vi "V_1.vi"() -> ()   [LabVIEW 2014]
uses:
  <vilib>/LabVIEW Interface for Arduino/Type Defs/Board Type.ctl
  <vilib>/LabVIEW Interface for Arduino/Type Defs/Connection Type.ctl
  <vilib>/LabVIEW Interface for Arduino/Type Defs/Pin Mode.ctl
  <vilib>/LabVIEW Interface for Arduino/LabVIEW Interface for Arduino.lvlib
panel:
  in  "Left":bool caption="Right"
  in  "Right":bool
  in  "VISA resource":refnum<visa-resource-name>
  in  "?":bool
  in  "Forward":bool
  in  "Backward":bool
  in  "Dial":dbl(knob) scale=0.0..255.0
  out "Speed":dbl(knob) scale=0.0..100.0
  # "ROBOT DIRECTION CONTROL AND SPEED CONTROL"
  # "VATSAL SHAH                       \nINDUS UNIVERSITY"
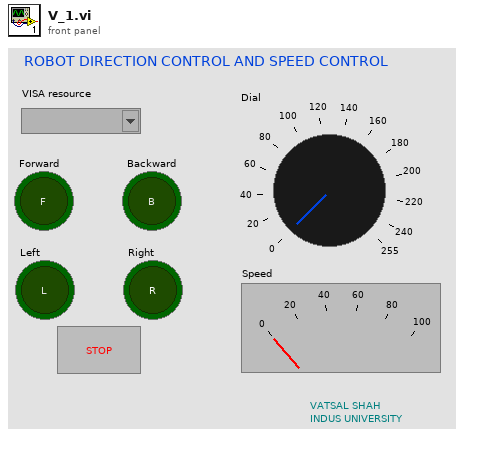
[diagram p1: front panel]
types:
  T1 = typedef "LabVIEW Interface for Arduino.lvlib/Connection Type.ctl" = enum8{"USB / Serial", "XBEE", "BlueSmirf (Bluetooth)"}
  T2 = typedef "LabVIEW Interface for Arduino.lvlib/Board Type.ctl" = enum16{"Uno", "Dimuelanove w/Atmega 328", "Mega 2560"}
  T3 = typedef "LabVIEW Interface for Arduino.lvlib/Arduino Resource.ctl" = cluster{"VISA resource":refnum<visa-resource-name>, "Board Type":T2, "Connection Type":enum8{"USB / Serial"}, "Bytes Per Packet (15)":u8}
  T4 = typedef "LabVIEW Interface for Arduino.lvlib/Pin Mode.ctl" = enum8{"Input", "Output"}
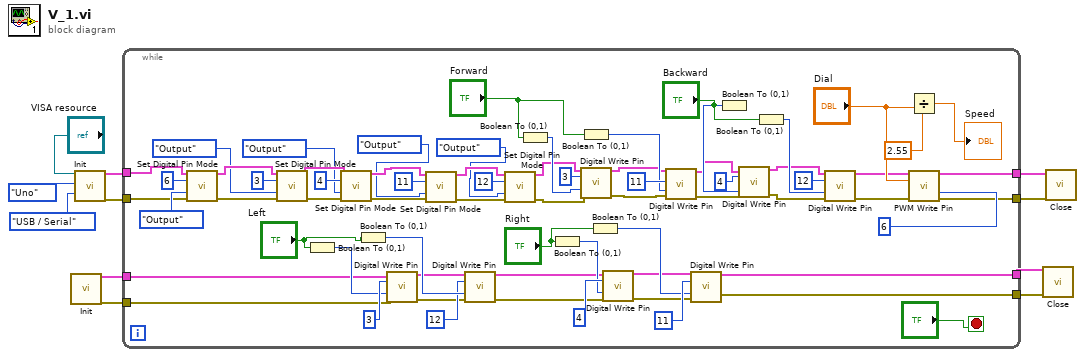
[diagram p0: block diagram]
diagram:
  n1 = call <vilib>:"Init.vi"() -> ("Arduino Resource"=w4:T3, "error out"=w3:errorcluster)  [unwired: 18 in]
  n2 = call <vilib>:"Init.vi"("VISA resource"="VISA resource", "Board Type (Uno)"=Board_Type."Uno", "Connection Type (USB/Serial)"=Connection_Type."USB / Serial") -> ("Arduino Resource"=w9:T3, "error out"=w10:errorcluster)  [unwired: 15 in]
  n3 = while {
    tunnel: w9 -> [w54]
    tunnel: w10 -> [w55]
    tunnel: [w66] -> w6
    tunnel: [w65] -> w5
    tunnel: w4 -> [w22]
    tunnel: w3 -> [w21]
    tunnel: [w13] -> w2
    tunnel: [w12] -> w1
    stop <- "?" stop-if-true
    n4 = call <vilib>:"Set Digital Pin Mode.vi"("Arduino Resource"=w54, "Digital I/O Pin"=u8 6, "Pin Mode (Input)"=Pin_Mode."Output", "error in"=w55) -> ("Arduino Resource"=w75:T3, "error out"=w74:errorcluster)  [unwired: 10 in]
    n5 = call <vilib>:"Set Digital Pin Mode.vi"("Arduino Resource"=w75, "Digital I/O Pin"=u8 3, "Pin Mode (Input)"=Pin_Mode."Output", "error in"=w74) -> ("Arduino Resource"=w57:T3, "error out"=w58:errorcluster)  [unwired: 10 in]
    n6 = Boolean To (0,1)(Boolean="Left") -> (0, 1=w53:i16)
    n7 = call <vilib>:"Set Digital Pin Mode.vi"("Arduino Resource"=w57, "Digital I/O Pin"=u8 4, "Pin Mode (Input)"=Pin_Mode."Output", "error in"=w58) -> ("Arduino Resource"=w44:T3, "error out"=w43:errorcluster)  [unwired: 10 in]
    n8 = Boolean To (0,1)(Boolean="Left") -> (0, 1=w50:i16)
    n9 = call <vilib>:"Digital Write Pin.vi"("Arduino Resource"=w22, "Digital I/O Pin (0)"=u8 3, "Value (0)"=w53, "error in"=w21) -> ("Arduino Resource"=w19:T3, "error out"=w18:errorcluster)  [unwired: 10 in]
    n10 = call <vilib>:"Set Digital Pin Mode.vi"("Arduino Resource"=w44, "Digital I/O Pin"=u8 11, "Pin Mode (Input)"=Pin_Mode."Output", "error in"=w43) -> ("Arduino Resource"=w42:T3, "error out"=w41:errorcluster)  [unwired: 10 in]
    n11 = call <vilib>:"Digital Write Pin.vi"("Arduino Resource"=w19, "Digital I/O Pin (0)"=u8 12, "Value (0)"=w50, "error in"=w18) -> ("Arduino Resource"=w17:T3, "error out"=w16:errorcluster)  [unwired: 10 in]
    n12 = call <vilib>:"Set Digital Pin Mode.vi"("Arduino Resource"=w42, "Digital I/O Pin"=u8 12, "Pin Mode (Input)"=Pin_Mode."Output", "error in"=w41) -> ("Arduino Resource"=w40:T3, "error out"=w39:errorcluster)  [unwired: 10 in]
    n13 = Boolean To (0,1)(Boolean="Forward") -> (0, 1=w46:i16)
    n14 = Boolean To (0,1)(Boolean="Right") -> (0, 1=w23:i16)
    n15 = Boolean To (0,1)(Boolean="Forward") -> (0, 1=w37:i16)
    n16 = call <vilib>:"Digital Write Pin.vi"("Arduino Resource"=w40, "Digital I/O Pin (0)"=u8 3, "Value (0)"=w46, "error in"=w39) -> ("Arduino Resource"=w35:T3, "error out"=w36:errorcluster)  [unwired: 10 in]
    n17 = Boolean To (0,1)(Boolean="Right") -> (0, 1=w24:i16)
    n18 = call <vilib>:"Digital Write Pin.vi"("Arduino Resource"=w17, "Digital I/O Pin (0)"=u8 4, "Value (0)"=w23, "error in"=w16) -> ("Arduino Resource"=w15:T3, "error out"=w14:errorcluster)  [unwired: 10 in]
    n19 = call <vilib>:"Digital Write Pin.vi"("Arduino Resource"=w35, "Digital I/O Pin (0)"=u8 11, "Value (0)"=w37, "error in"=w36) -> ("Arduino Resource"=w33:T3, "error out"=w32:errorcluster)  [unwired: 10 in]
    n20 = call <vilib>:"Digital Write Pin.vi"("Arduino Resource"=w15, "Digital I/O Pin (0)"=u8 11, "Value (0)"=w24, "error in"=w14) -> ("Arduino Resource"=w13:T3, "error out"=w12:errorcluster)  [unwired: 10 in]
    n21 = Boolean To (0,1)(Boolean="Backward") -> (0, 1=w70:i16)
    n22 = call <vilib>:"Digital Write Pin.vi"("Arduino Resource"=w33, "Digital I/O Pin (0)"=u8 4, "Value (0)"=w70, "error in"=w32) -> ("Arduino Resource"=w31:T3, "error out"=w30:errorcluster)  [unwired: 10 in]
    n23 = Boolean To (0,1)(Boolean="Backward") -> (0, 1=w64:i16)
    n24 = call <vilib>:"Digital Write Pin.vi"("Arduino Resource"=w31, "Digital I/O Pin (0)"=u8 12, "Value (0)"=w64, "error in"=w30) -> ("Arduino Resource"=w27:T3, "error out"=w26:errorcluster)  [unwired: 10 in]
    n25 = Divide(x="Dial", y=2.55) -> (x/y=→"Speed":dbl)
    n26 = call <vilib>:"PWM Write Pin.vi"("Arduino Resource"=w27, "Duty Cycle (0 - 255)"="Dial", "PWM Pin (3)"=u8 6, "error in"=w26) -> ("Arduino Resource"=w66:T3, "error out"=w65:errorcluster)  [unwired: 10 in]
  }
  n27 = call <vilib>:"Close.vi"("Arduino Resource"=w2, "error in"=w1) -> ()  [unwired: 13 in, 1 out]
  n28 = call <vilib>:"Close.vi"("Arduino Resource"=w6, "error in"=w5) -> ()  [unwired: 13 in, 1 out]
